vi "Write Set Selected Color.vi"(8 "error in (no error)":errorcluster, 10 "Selected Color":u32(colorbox), 11 "ColorSelector in":refnum<class "ColorSelector.lvclass">) -> (0 "error out":errorcluster, 3 "ColorSelector (dup)":refnum<class "ColorSelector.lvclass">)   [LabVIEW 2015, in "ColorSelector.lvclass"]
doc: "This Property VI is used in the owning VI as a Property Node to set the selected color of the <b>ColorSelector QControl</b>.\n<b> </b> <b> </b>\n©2017 Q Software Innovations, LLC (QSI)\nwritten by Quentin Alldredge\nproduced in LabVIEW 2015\n\nsupport@qsoftwareinnovations.com\nwww.qsoftwareinnovations.com\n\nAll rights reserved.\n\nRedistribution and use in source and binary forms, with or without modification, are permitted provided that the following conditions are met:\n\n * Redistributions of source code must retain the above copyright notice, this list of conditions and the following disclaimer.\n * Redistributions in binary form must reproduce the above copyright notice, this list of conditions and the following disclaimer in the documentation and/or other materials provided with the distribution.\n * Neither the name of Q Software Innovations, LLC. nor the names of its contributors may be used to endorse or promote products derived from this software without specific prior written permission.\n\nTHIS SOFTWARE IS PROVIDED BY THE COPYRIGHT HOLDERS AND CONTRIBUTORS \"AS IS\" AND ANY EXPRESS OR IMPLIED WARRANTIES, INCLUDING, BUT NOT LIMITED TO, THE IMPLIED WARRANTIES OF MERCHANTABILITY AND FITNESS FOR A PARTICULAR PURPOSE ARE DISCLAIMED. IN NO EVENT SHALL THE COPYRIGHT OWNER OR CONTRIBUTORS BE LIABLE FOR ANY DIRECT, INDIRECT, INCIDENTAL, SPECIAL, EXEMPLARY, OR CONSEQUENTIAL DAMAGES (INCLUDING, BUT NOT LIMITED TO, PROCUREMENT OF SUBSTITUTE GOODS OR SERVICES; LOSS OF USE, DATA, OR PROFITS; OR BUSINESS INTERRUPTION) HOWEVER CAUSED AND ON ANY THEORY OF LIABILITY, WHETHER IN CONTRACT, STRICT LIABILITY, OR TORT (INCLUDING NEGLIGENCE OR OTHERWISE) ARISING IN ANY WAY OUT OF THE USE OF THIS SOFTWARE, EVEN IF ADVISED OF THE POSSIBILITY OF SUCH DAMAGE."
uses:
  ColorSelector.lvclass
  ColorSelector.lvclass/ColorSelector.ctl
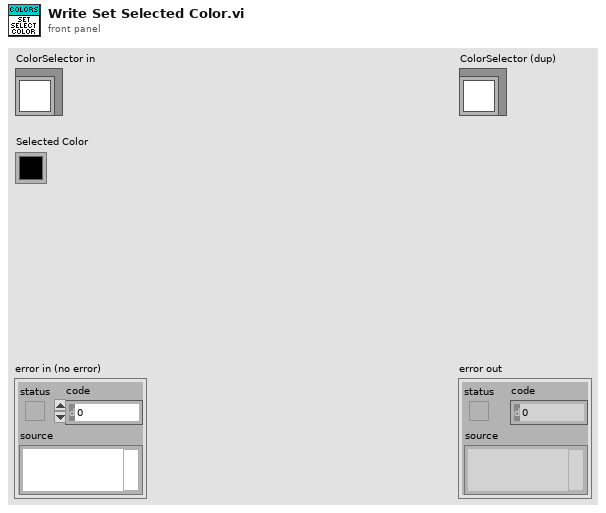
[diagram p1: front panel]
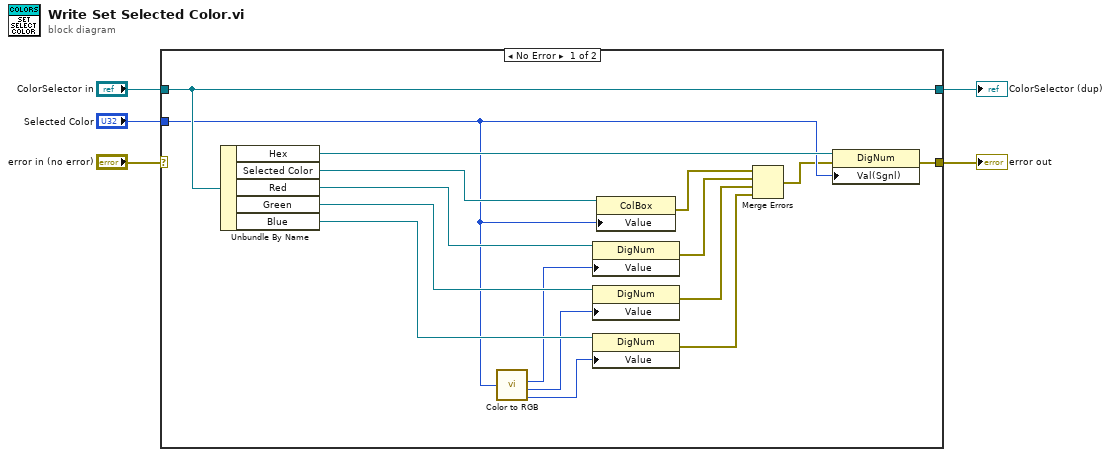
[diagram p0: block diagram]
diagram:
  n1 = case shown="No Error" "error in (no error)" {
    selector: "error in (no error)" -> [_ w23]
    tunnel: [w6 w23] -> w4
    tunnel: [w21 w22] -> w2
    tunnel: "ColorSelector in" -> [w21 w22]
    tunnel: "Selected Color" -> [w12 _]
    frame No Error {
      n2 = Unbundle By Name(w21) -> ("Hex"=w20:refnum<vi>, "Selected Color"=w13:refnum<vi>, "Red"=w19:refnum<vi>, "Green"=w18:refnum<vi>, "Blue"=w17:refnum<vi>)
      n3 = call <vilib>:"Color to RGB.vi"("Color"=w12) -> ("R"=w14:u8, "G"=w15:u8, "B"=w16:u8)  [unwired: 1 out]
      n4 = property class="DigNum"(reference=w19, "Value"=w14) -> (error out=w10:errorcluster)  [unwired: 1 in, 1 out]
      n5 = property class="DigNum"(reference=w18, "Value"=w15) -> (error out=w9:errorcluster)  [unwired: 1 in, 1 out]
      n6 = property class="DigNum"(reference=w17, "Value"=w16) -> (error out=w8:errorcluster)  [unwired: 1 in, 1 out]
      n7 = property class="ColBox"(reference=w13, "Value"=w12) -> (error out=w11:errorcluster)  [unwired: 1 in, 1 out]
      n8 = Merge Errors(w11, w10, w9, w8) -> (w7:errorcluster)
      n9 = property class="DigNum"(reference=w20, error in=w7, "Val(Sgnl)"=w12) -> (error out=w6:errorcluster)  [unwired: 1 out]
    }
    frame Error {
    }
  }
  "error out" <- w4
  "ColorSelector (dup)" <- w2
